vi "setUp.vi"(8 "error in (no error)":errorcluster, 11 "reference in":refnum<class "Interface Framework Multiple Objects.lvclass">) -> (0 "error out":errorcluster, 3 "reference in":refnum<class "Interface Framework Multiple Objects.lvclass">)   [LabVIEW 2009, in "Interface Framework Multiple Objects.lvclass"]
doc: "setUp runs prior to the test method during test execution. Use this method to initialize any object data required by your tests."
uses:
  Interface Framework Multiple Objects.lvclass
  Numeric Test Object/Numeric Test Object.lvclass
  Interface Framework Multiple Objects.lvclass/Interface Framework Multiple Objects.ctl
  <vilib>/addons/_JKI Toolkits/VI Tester/TestCase.llb/TestCase.lvclass
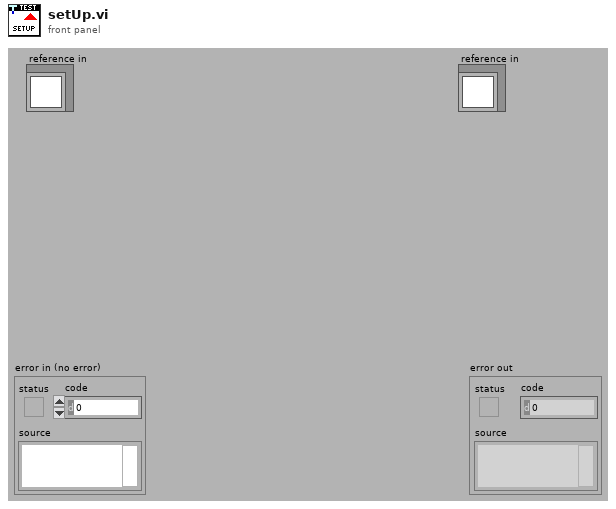
[diagram p1: front panel]
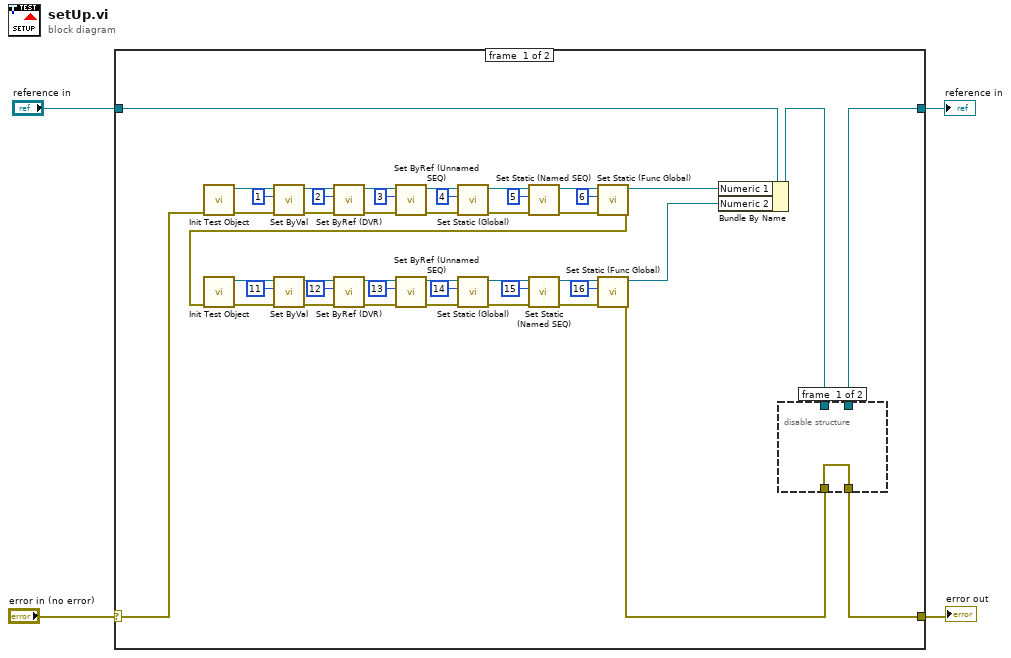
[diagram p0: block diagram]
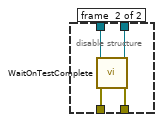
[diagram p2: hidden frame]
diagram:
  n1 = case shown="No Error" "error in (no error)" {
    selector: "error in (no error)" -> [w28 w57]
    tunnel: [w48 w57] -> w3
    tunnel: [w49 w56] -> w1
    tunnel: "reference in" -> [w47 w56]
    frame #0 {
      n2 = call "Init Test Object.vi"("error in (no error)"=w28) -> ("error out"=w46:errorcluster, "Numeric out"=w45:refnum<class "Numeric Test Object.lvclass">)  [unwired: 9 in]
      n3 = call-dynamic "Set ByVal.vi"("error in (no error)"=w46, "Int"=1, "Numeric in"=w45) -> ("error out"=w34:errorcluster, "Numeric out"=w29:refnum<class "Numeric Test Object.lvclass">)  [unwired: 7 in]
      n4 = call-dynamic "Set ByRef (DVR).vi"("error in (no error)"=w34, "Int"=2, "Numeric in"=w29) -> ("error out"=w35:errorcluster, "Numeric out"=w30:refnum<class "Numeric Test Object.lvclass">)  [unwired: 7 in]
      n5 = call-dynamic "Set ByRef (Unnamed SEQ).vi"("error in (no error)"=w35, "Int"=3, "Numeric in"=w30) -> ("error out"=w37:errorcluster, "Numeric out"=w36:refnum<class "Numeric Test Object.lvclass">)  [unwired: 7 in]
      n6 = call-dynamic "Set Static (Global).vi"("error in (no error)"=w37, "Int"=4, "Numeric in"=w36) -> ("error out"=w43:errorcluster, "Numeric out"=w39:refnum<class "Numeric Test Object.lvclass">)  [unwired: 7 in]
      n7 = call-dynamic "Set Static (Named SEQ).vi"("error in (no error)"=w43, "Int"=5, "Numeric in"=w39) -> ("error out"=w44:errorcluster, "Numeric out"=w41:refnum<class "Numeric Test Object.lvclass">)  [unwired: 7 in]
      n8 = call-dynamic "Set Static (Func Global).vi"("error in (no error)"=w44, "Int"=6, "Numeric in"=w41) -> ("error out"=w9:errorcluster, "Numeric out"=w6:refnum<class "Numeric Test Object.lvclass">)  [unwired: 7 in]
      n9 = call "Init Test Object.vi"("error in (no error)"=w9) -> ("error out"=w10:errorcluster, "Numeric out"=w11:refnum<class "Numeric Test Object.lvclass">)  [unwired: 9 in]
      n10 = call-dynamic "Set ByVal.vi"("error in (no error)"=w10, "Int"=11, "Numeric in"=w11) -> ("error out"=w22:errorcluster, "Numeric out"=w27:refnum<class "Numeric Test Object.lvclass">)  [unwired: 7 in]
      n11 = call-dynamic "Set ByRef (DVR).vi"("error in (no error)"=w22, "Int"=12, "Numeric in"=w27) -> ("error out"=w21:errorcluster, "Numeric out"=w26:refnum<class "Numeric Test Object.lvclass">)  [unwired: 7 in]
      n12 = call-dynamic "Set ByRef (Unnamed SEQ).vi"("error in (no error)"=w21, "Int"=13, "Numeric in"=w26) -> ("error out"=w19:errorcluster, "Numeric out"=w20:refnum<class "Numeric Test Object.lvclass">)  [unwired: 7 in]
      n13 = call-dynamic "Set Static (Global).vi"("error in (no error)"=w19, "Int"=14, "Numeric in"=w20) -> ("error out"=w13:errorcluster, "Numeric out"=w17:refnum<class "Numeric Test Object.lvclass">)  [unwired: 7 in]
      n14 = call-dynamic "Set Static (Named SEQ).vi"("error in (no error)"=w13, "Int"=15, "Numeric in"=w17) -> ("error out"=w12:errorcluster, "Numeric out"=w15:refnum<class "Numeric Test Object.lvclass">)  [unwired: 7 in]
      n15 = call-dynamic "Set Static (Func Global).vi"("error in (no error)"=w12, "Int"=16, "Numeric in"=w15) -> ("error out"=w8:errorcluster, "Numeric out"=w5:refnum<class "Numeric Test Object.lvclass">)  [unwired: 7 in]
      n16 = Bundle By Name(cluster=w47, "Numeric 1"=w6, "Numeric 2"=w5) -> (w7:refnum<class "Interface Framework Multiple Objects.lvclass">)
      n17 = disable-structure shown="Enabled" {
        disable-tunnel: w7 -> [w51 w55]
        disable-tunnel: [w51 w54] -> w49
        disable-tunnel: w8 -> [w50 w53]
        disable-tunnel: [w50 w52] -> w48
        frame #0 {
          # "If no references opened by\nsetUp then enable this frame"
        }
        frame #1 {
          n18 = call <vilib>:"WaitOnTestComplete.vi"("error in (no error)"=w53, "TestCase in"=w55) -> ("error out"=w52:errorcluster, "TestCase out"=w54:refnum<class "Interface Framework Multiple Objects.lvclass">)  [unwired: 8 in]
        }
      }
    }
    frame #1 {
    }
  }
  "error out" <- w3
  "reference in" <- w1
